vi "向导型多页面对话框.vi"() -> ()   [LabVIEW 2013]
panel:
  in  "OVERVIEW_PRE":bool
  in  "OVERVIEW_NEXT":bool
  in  "OVERVIEW_Exit":bool
  out "OVERVIEW_Tab":enum32{"Page1", "Page2", "Page3", "Page4"}(tab) caption="MD_Tab"
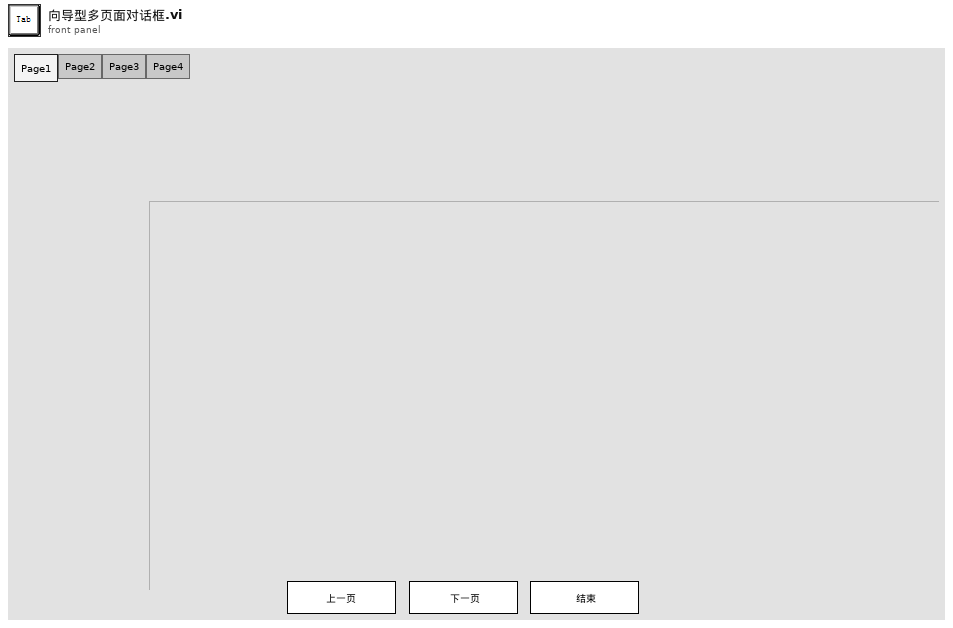
[diagram p1: front panel]
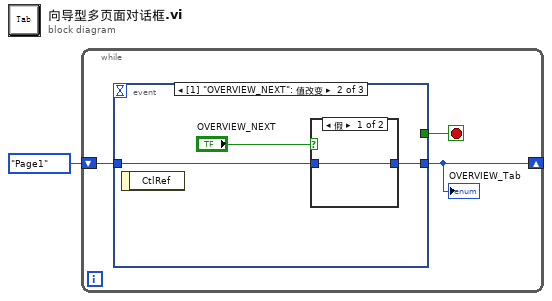
[diagram p0: block diagram]
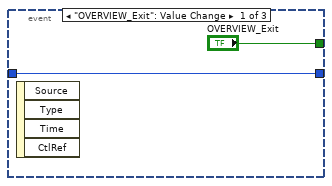
[diagram p2: hidden frame]
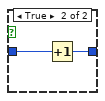
[diagram p3: hidden frame]
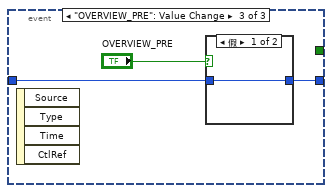
[diagram p4: hidden frame]
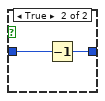
[diagram p5: hidden frame]
diagram:
  n1 = while {
    shift-right: [w2] -> _
    shift-left: enum32{"Page1", "Page2", "Page3", "Page4"}."Page1" ("OVERVIEW_Tab") -> [w3]
    stop <- w4 stop-if-true
    n2 = event shown="[1] \"OVERVIEW_NEXT\": 值改变" {
      selector: _ -> [_ _ _]
      dyn-events: _ -> [_ _ _]
      timeout: _ -> [_ _ _]
      tunnel: ["OVERVIEW_Exit" _ _] -> w4
      tunnel: w3 -> [w5 w9 w15]
      tunnel: [w5 w8 w14] -> w2
      event "OVERVIEW_Exit": Value Change {
        n3 = event-data() -> ()  [unwired: 1 in, 4 out]
      }
      event "OVERVIEW_NEXT": Value Change {
        n4 = event-data() -> ()  [unwired: 1 in, 1 out]
        n5 = case shown="假" "OVERVIEW_NEXT" {
          tunnel: w9 -> [w10 w12]
          tunnel: [w10 w11] -> w8
          frame False {
          }
          frame True {
            n6 = Increment(x=w12) -> (x+1=w11:enum32{"Page1", "Page2", "Page3", "Page4"})
          }
        }
      }
      event "OVERVIEW_PRE": Value Change {
        n7 = event-data() -> ()  [unwired: 1 in, 4 out]
        n8 = case shown="假" "OVERVIEW_PRE" {
          tunnel: w15 -> [w16 w18]
          tunnel: [w16 w17] -> w14
          frame False {
          }
          frame True {
            n9 = Decrement(x=w18) -> (x-1=w17:enum32{"Page1", "Page2", "Page3", "Page4"})
          }
        }
      }
    }
    "OVERVIEW_Tab" <- w2
  }
